vi "Logger.HandleNAme.vi"(11 "String":string) -> (1 "SerialNo":string, 2 "Variant":string, 3 "System":string)   [LabVIEW 2016]
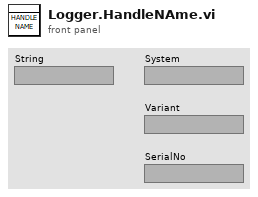
[diagram p1: front panel]
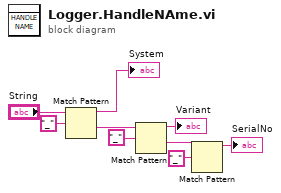
[diagram p0: block diagram]
diagram:
  n1 = Match Pattern(string="String", regular expression="_") -> (before substring=→"System":string, after substring=w4:string)  [unwired: 1 in, 2 out]
  n2 = Match Pattern(string=w4, regular expression="_") -> (before substring=→"Variant":string, after substring=w7:string)  [unwired: 1 in, 2 out]
  n3 = Match Pattern(string=w7, regular expression="_") -> (before substring=→"SerialNo":string)  [unwired: 1 in, 3 out]
